vi "Ball Intake Logging.vi"   [LabVIEW 2016]
uses:
  Robot Global Data.vi
  Ball Intake Logging Values.vi
types:
  T1 = typedef "WPI_DriverStationRobotMode2.ctl" = enum16{"Autonomous Disabled", "Autonomous Enabled", "Teleop Disabled", "Teleop Enabled", "Disconnected", "Finish", "Test Disabled", "Test Enabled", "Emergency Stopped"}
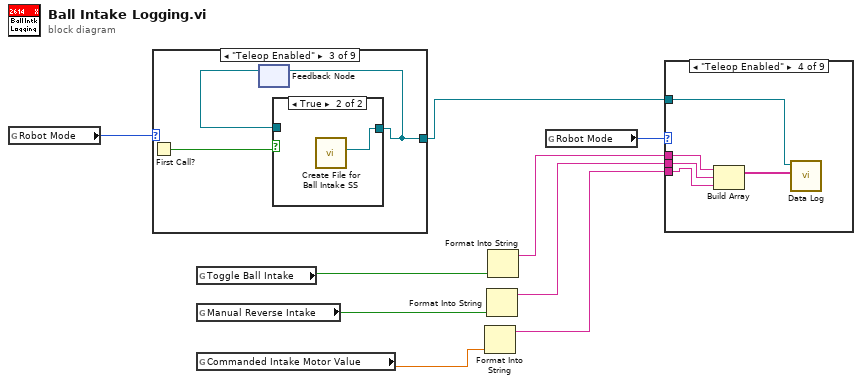
[diagram p0: block diagram]
diagram:
  n1 = global read "Robot Global Data.vi" "Robot Mode"() -> (w9:T1)
  n2 = case shown="\"Teleop Enabled\"" w9 {
    tunnel: [_ _ w10 _ _ _ _ _ _] -> w4
    frame "Autonomous Enabled" {
    }
    frame "Teleop Disabled", Default {
    }
    frame "Teleop Enabled" {
      n3 = First Call?() -> (First Call?: T/F=w12:bool)
      n4 = feedback #1() -> (w11:refnum<file>)  [unwired: 1 in]
      n5 = case shown="True" w12 {
        tunnel: [w13 w14] -> w10
        tunnel: w11 -> [w13 _]
        frame False {
        }
        frame True {
          n6 = call "Create File for Ball Intake SS.vi"() -> ("File Reference Out"=w14:refnum<file>)  [unwired: 11 in]
        }
      }
      n7 = feedback-in #1(w10) -> ()
    }
    frame "Disconnected" {
    }
    frame "Finish" {
    }
    frame "Test Disabled" {
    }
    frame "Test Enabled" {
    }
    frame "Emergency Stopped" {
    }
    frame "Autonomous Disabled" {
    }
  }
  n8 = global read "Ball Intake Logging Values.vi" "Toggle Ball Intake"() -> (w3:bool)
  n9 = global read "Ball Intake Logging Values.vi" "Manual Reverse Intake"() -> (w2:bool)
  n10 = global read "Ball Intake Logging Values.vi" "Commanded Intake Motor Value"() -> (w1:dbl)
  n11 = Format Into String(w1) -> (resulting string=w6:string)  [unwired: 3 in, 1 out]
  n12 = Format Into String(w2) -> (resulting string=w7:string)  [unwired: 3 in, 1 out]
  n13 = Format Into String(w3) -> (resulting string=w8:string)  [unwired: 3 in, 1 out]
  n14 = global read "Robot Global Data.vi" "Robot Mode"() -> (w5:T1)
  n15 = case shown="\"Teleop Enabled\"" w5 {
    tunnel: w8 -> [_ _ _ w18 _ _ _ _ _]
    tunnel: w7 -> [_ _ _ w17 _ _ _ _ _]
    tunnel: w6 -> [_ _ _ w16 _ _ _ _ _]
    tunnel: w4 -> [_ _ _ w15 _ _ _ _ _]
    frame "Autonomous Disabled", Default {
    }
    frame "Autonomous Enabled" {
    }
    frame "Teleop Disabled" {
    }
    frame "Teleop Enabled" {
      n16 = Build Array(w18, w17, w16) -> (w19:string[])
      n17 = call "Data Log.vi"("Data In"=w19, "File Reference In"=w15) -> ()  [unwired: 9 in, 1 out]
    }
    frame "Disconnected" {
    }
    frame "Finish" {
    }
    frame "Test Disabled" {
    }
    frame "Test Enabled" {
    }
    frame "Emergency Stopped" {
    }
  }
